vi "Time_171213.vi"(11 "TimeIn":T1) -> (2 "TimeOut":string, 3 "TimeOut":T1)   [LabVIEW 2016]
uses:
  <vilib>/Utility/miscctls.llb/LVDateTimeRec.ctl
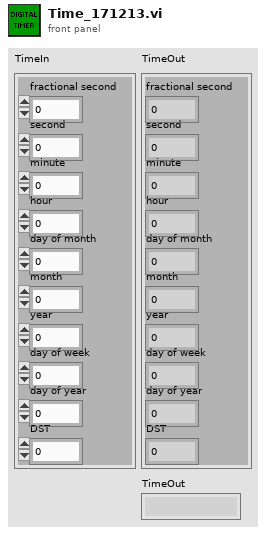
[diagram p1: front panel]
types:
  T1 = typedef "LVDateTimeRec.ctl" = cluster{"fractional second":dbl, "second":i32, "minute":i32, "hour":i32, "day of month":i32, "month":i32, "year":i32, "day of week":i32, "day of year":i32, "DST":i32}
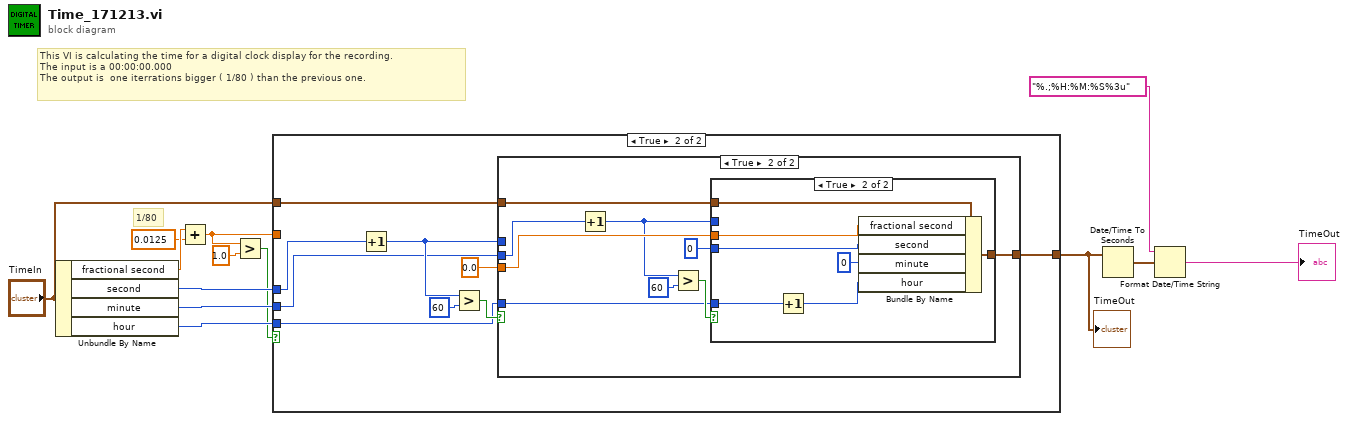
[diagram p0: block diagram]
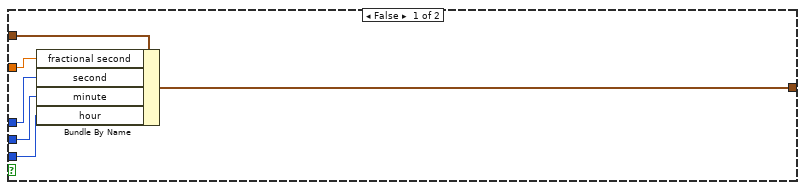
[diagram p2: hidden frame]
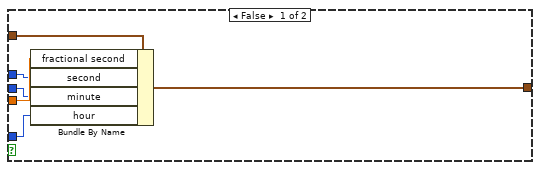
[diagram p3: hidden frame]
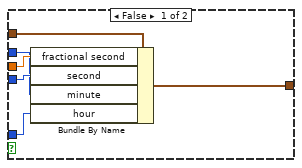
[diagram p4: hidden frame]
diagram:
  # "This VI is calculating the time for a digital clock display for the recording.\nThe input is a 00:00:00.000\nThe output is  one iterrations bigger ( 1/80 ) than the previous one."
  # "1/80"
  n1 = Unbundle By Name("TimeIn") -> ("fractional second"=w6:dbl, "second"=w11:i32, "minute"=w12:i32, "hour"=w13:i32)
  n2 = Add(x=w6, y=0.0125) -> (x+y=w9:dbl)
  n3 = Greater?(x=w9, y=1.0) -> (0:w5:bool)
  n4 = case shown="True" w5 {
    tunnel: "TimeIn" -> [w19 w27]
    tunnel: [w18 w28] -> w10
    tunnel: w9 -> [w17 _]
    tunnel: w11 -> [w16 w24]
    tunnel: w12 -> [w15 w22]
    tunnel: w13 -> [w14 w21]
    frame False {
      n5 = Bundle By Name(cluster=w19, "fractional second"=w17, "second"=w16, "minute"=w15, "hour"=w14) -> (w18:T1)
    }
    frame True {
      n6 = Increment(x=w24) -> (x+1=w23:i32)
      n7 = Greater?(x=w23, y=60) -> (0:w26:bool)
      n8 = case shown="True" w26 {
        tunnel: [w34 w39] -> w28
        tunnel: w27 -> [w33 w40]
        tunnel: 0.0 ("y") -> [w32 w38]
        tunnel: w23 -> [w31 _]
        tunnel: w22 -> [w30 w43]
        tunnel: w21 -> [w29 w37]
        frame False {
          n9 = Bundle By Name(cluster=w33, "fractional second"=w32, "second"=w31, "minute"=w30, "hour"=w29) -> (w34:T1)
        }
        frame True {
          n10 = Increment(x=w43) -> (x+1=w36:i32)
          n11 = Greater?(x=w36, y=60) -> (0:w41:bool)
          n12 = case shown="True" w41 {
            tunnel: w40 -> [w49 w56]
            tunnel: [w48 w55] -> w39
            tunnel: w38 -> [w47 w54]
            tunnel: 0 ("y") -> [w46 w53]
            tunnel: w37 -> [w44 w52]
            tunnel: w36 -> [w45 _]
            frame False {
              n13 = Bundle By Name(cluster=w49, "fractional second"=w47, "second"=w46, "minute"=w45, "hour"=w44) -> (w48:T1)
            }
            frame True {
              n14 = Increment(x=w52) -> (x+1=w51:i32)
              n15 = Bundle By Name(cluster=w56, "fractional second"=w54, "second"=w53, "minute"=0 ("y"), "hour"=w51) -> (w55:T1)
            }
          }
        }
      }
    }
  }
  "TimeOut" <- w10
  n16 = Date/Time To Seconds(2:w10) -> (0:w4:timestamp)  [unwired: 1 in]
  n17 = Format Date/Time String(time format string (%c)="%.;%H:%M:%S%3u", seconds (now)=w4) -> (date/time string=→"TimeOut":string)  [unwired: 1 in]
